vi "Teleop.vi"(10 "Match Info":T1={"Autonomous Elapsed Seconds"=0.0, "TeleOp Elapsed Seconds"=0.0, "Disabled Elapsed Seconds"=0.0, "Visited Autonomous"=FALSE, "Visited TeleOp"=FALSE, "Visited Disabled"=FALSE, "Autonomous Settings"={"Autonomous Style"=enum."Independent", "VI Refnum"=refnum}}, 11 "Call Context":T2) -> ()   [LabVIEW 2016]
doc: "This VI is called for each enabled TeleOp packet received from the DS. It is typically used to read from joysticks and other inputs and update I/O or setpoints for timed control loops. It should complete and return within 20 milliseconds or risk missing DS packets."
uses:
  <vilib>/Rock Robotics/WPI/DriverStation/WPI_DriverStationDerivedRobotMode.ctl
  <vilib>/Rock Robotics/WPI/DriverStation/WPI_DriverStationMatch Info.ctl
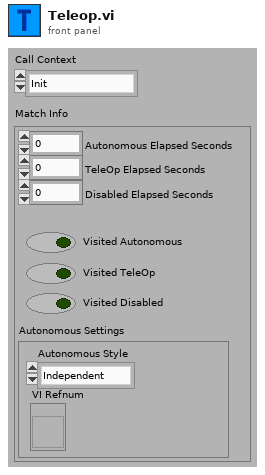
[diagram p1: front panel]
types:
  T1 = typedef "WPI_DriverStationMatch Info.ctl" = cluster{"Autonomous Elapsed Seconds":dbl, "TeleOp Elapsed Seconds":dbl, "Disabled Elapsed Seconds":dbl, "Visited Autonomous":bool, "Visited TeleOp":bool, "Visited Disabled":bool, "Autonomous Settings":cluster{"Autonomous Style":enum16{"Iterative", "Independent"}, "VI Refnum":refnum<vi>}}
  T2 = typedef "WPI_DriverStationDerivedRobotMode.ctl" = enum16{"Init", "Execute", "Stop"}
  T3 = cluster{"A":bool, "B":bool, "X":bool, "Y":bool, "LB":bool, "RB":bool, "Back":bool, "Start":bool, "LC":bool, "RC":bool, "LT":bool, "RT":bool}
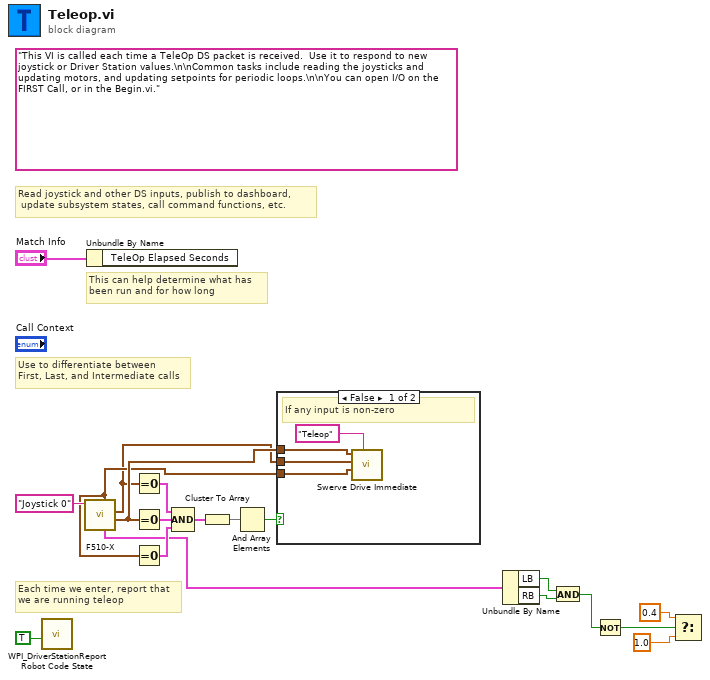
[diagram p0: block diagram]
diagram:
  (unwired) "This VI is called each time a TeleOp DS packet is received.  Use it to respond to new joystick or Driver Station values.\n\nCommon tasks include reading the joysticks and updating motors, and updating setpoints for periodic loops.\n\nYou can open I/O on the FIRST Call, or in the Begin.vi."
  # "Read joystick and other DS inputs, publish to dashboard,\n update subsystem states, call command functions, etc."
  # "Each time we enter, report that\nwe are running teleop"
  # "Use to differentiate between\nFirst, Last, and Intermediate calls"
  # "This can help determine what has\nbeen run and for how long"
  n1 = call <vilib>:"WPI_DriverStationReport Robot Code State.vi"("TeleOp"=TRUE ("Autonomous")) -> ()  [unwired: 10 in, 1 out]
  n2 = call "F510-X.vi"("refnum name"="Joystick 0") -> ("Right Stick"=w3:cluster{"X":dbl, "Y":dbl}, "Left Stick"=w1:cluster{"X":dbl, "Y":dbl}, "Buttons"=w4:T3, "Triggers"=w2:cluster{"Left":dbl, "Right":dbl})  [unwired: 4 in, 3 out]
  n3 = Unbundle By Name("Match Info") -> ()  [unwired: 1 out]
  n4 = Equal To 0?(x=w1) -> (x = 0?=w16:cluster{"X":bool, "Y":bool})
  n5 = Equal To 0?(x=w3) -> (x = 0?=w15:cluster{"X":bool, "Y":bool})
  n6 = Equal To 0?(x=w2) -> (x = 0?=w14:cluster{"Left":bool, "Right":bool})
  n7 = Compound Arithmetic op=AND(w16, w15, w14) -> (w13:cluster{bool, bool})
  n8 = Cluster To Array(cluster=w13) -> (array=w12:bool[])
  n9 = And Array Elements(Boolean array=w12) -> (logical AND=w11:bool)
  n10 = case shown="False" w11 {
    tunnel: w2 -> [w22 _]
    tunnel: w3 -> [w21 _]
    tunnel: w1 -> [w20 _]
    frame False {
      # "If any input is non-zero"
      n11 = call "Swerve Drive Immediate.vi"("Description"="Teleop", "Trigger Axes"=w22, "Face Joystick Axes"=w20, "Strafe Joystick Axes"=w21) -> ()  [unwired: 7 in, 1 out]
    }
    frame True {
      # "If all inputs are zero"
    }
  }
  n12 = Unbundle By Name(w4) -> ("LB"=w9:bool, "RB"=w8:bool)
  n13 = And(x=w9, y=w8) -> (x .and. y?=w10:bool)
  n14 = Not(x=w10) -> (.not. x?=w5:bool)
  n15 = Select(t=0.4 ("Slow Speed Multiplier"), s=w5, f=1.0 ("Default Speed Multiplier")) -> ()  [unwired: 1 out]
